vi "Close.vi"(8 "error in":errorcluster, 11 "Humidity Limit in":refnum<class "Humidity Limit.lvclass">) -> (0 "error out":errorcluster, 3 "Humidity Limit out":refnum<class "Humidity Limit.lvclass">)   [LabVIEW 2023, in "Humidity Limit.lvclass"]
uses:
  Humidity Limit.lvclass
  Parents/Limit/Limit.lvclass
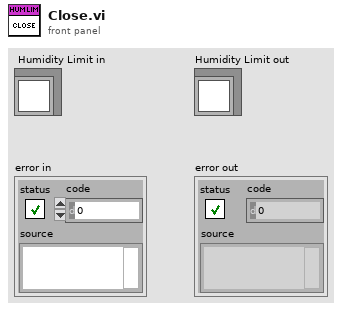
[diagram p1: front panel]
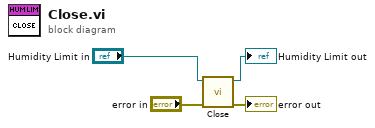
[diagram p0: block diagram]
diagram:
  n1 = call-parent "Close.vi"("error in"="error in", "Limit in"="Humidity Limit in") -> ("error out"=→"error out":errorcluster, "Limit out"=→"Humidity Limit out":refnum<class "Humidity Limit.lvclass">)  [unwired: 8 in]
